vi "DriveAngleHAdvanced.vi"(2 "Parameter String":string, 3 "Reinit":bool) -> (0 "Error Out":errorcluster, 1 "Increment":bool)   [LabVIEW 2020]
doc: "The swerve drive base will rotate about its center at a speed specified by the joystick command. This is a \"medium smart\" algorithm, the angle has to be within the specified range for a certain amount of time. Any complex or critical turns should be handled using either the Path Follower or auto-targeting. \n\nParameters:\n1. field-centric angle --> (deg) [0,360]\n2. error- the number of degrees on either side of the goal allowed --> (deg) [0,360]"
uses:
  SafeParser_Float.vi
  drivercommands.vi
  sensordata.vi
panel:
  in  "Time in Range (ms)":u32=1000
  in  "Plots?":bool
  out "Controller Summary":T1(graph)
  in  "PID Tuning Parameters":T2={"Kp"=0.01, "Ki"=0.01, "Kd"=9e-05, "N-Diff"=10, "N-Int"=20, "Int Error Window"=0.5, "Max Ouput"=1.0, "Min Output"=-1.0} {"Int Error Window" min=0.0; "N-Int" min=2; "N-Diff" min=2; "Kd" min=0.0; "Ki" min=0.0; "Kp" min=0.0}
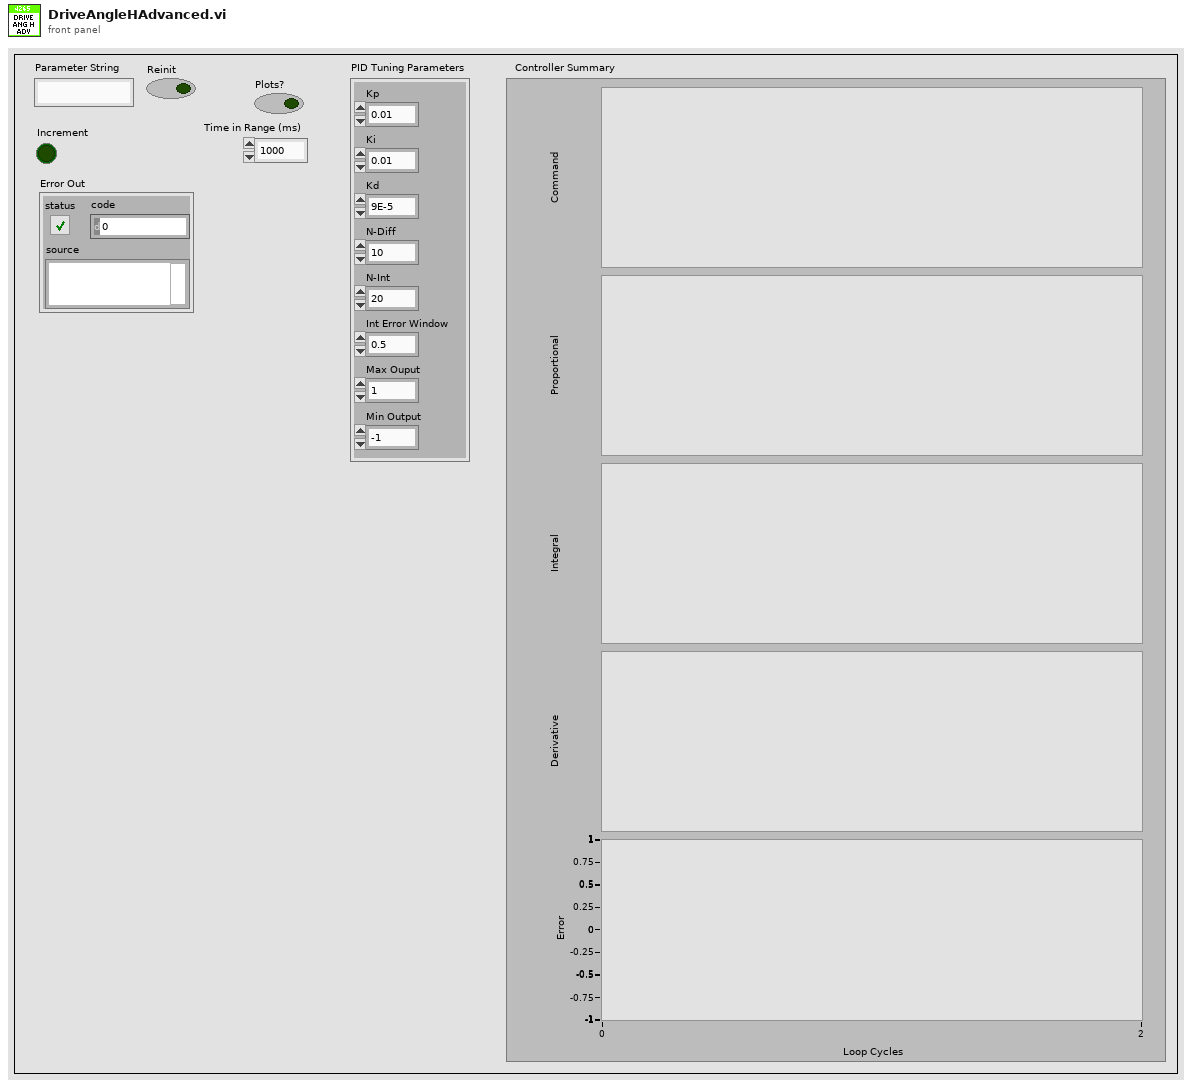
[diagram p1: front panel]
types:
  T1 = cluster{"Command":dbl, "Proportional":dbl, "Integral":dbl, "Derivative":dbl, "Goal":dbl}
  T2 = cluster{"Kp":dbl, "Ki":dbl, "Kd":dbl, "N-Diff":i32, "N-Int":i32, "Int Error Window":dbl, "Max Ouput":dbl, "Min Output":dbl}
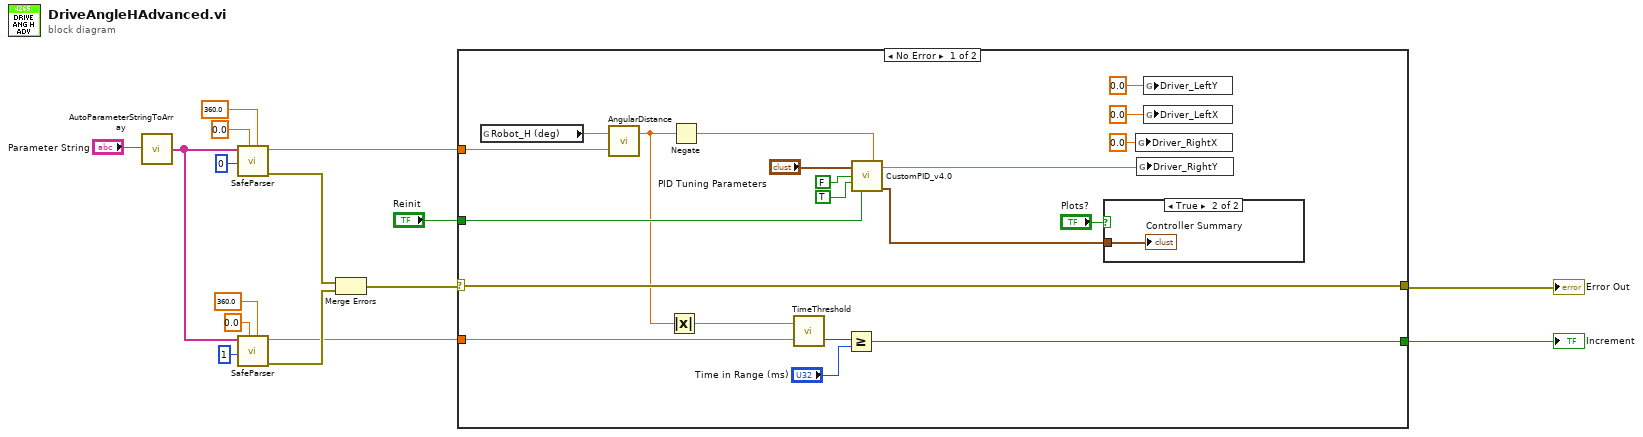
[diagram p0: block diagram]
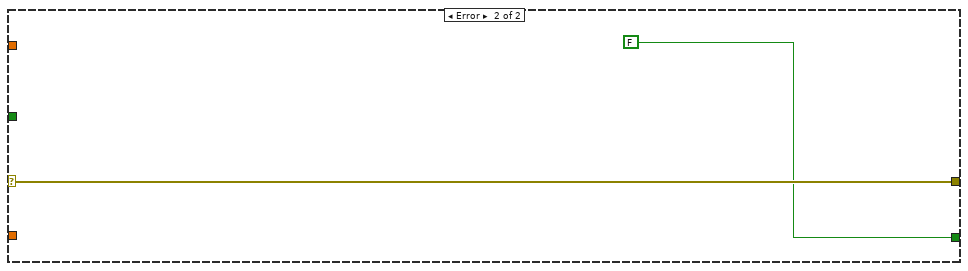
[diagram p3: hidden frame]
diagram:
  n1 = call "AutoParameterStringToArray.vi"("Parameter String"="Parameter String") -> ("Parsed Parameters"=w4:string[])
  n2 = call-poly "SafeParser.vi"("Maximum"=360.0, "Minimum"=0.0, "Array Index"=0 ("Parameter Index"), "String Array"=w4) -> ("Error Out"=w9:errorcluster, "Typecast  Value"=w7:dbl)  [unwired: 6 in]
  n3 = call-poly "SafeParser.vi"("Maximum"=360.0, "Minimum"=0.0, "Array Index"=1 ("Parameter Index"), "String Array"=w4) -> ("Error Out"=w8:errorcluster, "Typecast  Value"=w3:dbl)  [unwired: 6 in]
  n4 = Merge Errors(w9, w8) -> (w10:errorcluster)
  n5 = case shown="No Error" w10 {
    selector: w10 -> [w33 w39]
    tunnel: [w18 FALSE] -> w1
    tunnel: [w33 w39] -> w16
    tunnel: w7 -> [w32 _]
    tunnel: w3 -> [w19 _]
    tunnel: "Reinit" -> [w23 _]
    frame No Error {
      n6 = global read "sensordata.vi" "Robot_H (deg)"() -> (w22:dbl)
      n7 = call "AngularDistance.vi"("Goal Angle (deg) [0,360]"=w32, "Current Angle (deg) [-Inf,+Inf]"=w22) -> ("Signed Angular Distance (deg) [-180,+180]"=w21:dbl)  [unwired: 1 out]
      n8 = Absolute Value(x=w21) -> (abs(x)=w20:dbl)
      n9 = Negate(x=w21) -> (-x=w17:dbl)
      n10 = call "TimeThreshold.vi"("Threshold"=w19, "Current Value"=w20) -> ("Time Below Threshold (ms)"=w25:u32)  [unwired: 1 out]
      n11 = Greater Or Equal?(x=w25, y="Time in Range (ms)") -> (x >= y?=w18:bool)
      n12 = call "CustomPID_v4.0.vi"("PID Tuning Parameters"="PID Tuning Parameters", "Custom Error Calculation"=w17, "Reset on Goal Change ?"=FALSE, "Use Custom Error Calculation ?"=TRUE ("Reset on Goal Change ?"), "Reinit"=w23) -> ("Command"=w28:dbl, "Controller Summary"=w26:T1)  [unwired: 7 in, 2 out]
      n13 = case shown="True" "Plots?" {
        tunnel: w26 -> [_ w37]
        frame False {
        }
        frame True {
          "Controller Summary" <- w37
        }
      }
      n14 = global write "drivercommands.vi" "Driver_RightX"(0.0 ("Driver_RightX")) -> ()
      n15 = global write "drivercommands.vi" "Driver_RightY"(w28) -> ()
      n16 = global write "drivercommands.vi" "Driver_LeftY"(0.0 ("Driver_RightX")) -> ()
      n17 = global write "drivercommands.vi" "Driver_LeftX"(0.0 ("Driver_RightX")) -> ()
    }
    frame Error {
    }
  }
  "Increment" <- w1
  "Error Out" <- w16
